vi "setUp.vi"(8 "error in (no error)":errorcluster, 11 "reference in":refnum<class "Telemetry System Tests.lvclass">) -> (0 "error out":errorcluster, 3 "reference out":refnum<class "Telemetry System Tests.lvclass">)   [LabVIEW 2019, in "Telemetry System Tests.lvclass"]
doc: "setUp runs prior to the test method during test execution. Use this method to initialize any object data required by your tests."
uses:
  Telemetry System Tests.lvclass
  C:/Program Files (x86)/National Instruments/LabVIEW 2019/vi.lib/addons/_JKI Toolkits/VI Tester/TestCase.llb/TestCase.lvclass
  Telemetry System Tests.lvclass/Telemetry System Tests.ctl
  <vilib>/addons/_JKI Toolkits/VI Tester/TestCase.llb/TestCase.lvclass
  Telemetry Test Utilities/Telemetry Test Utilities.lvlib
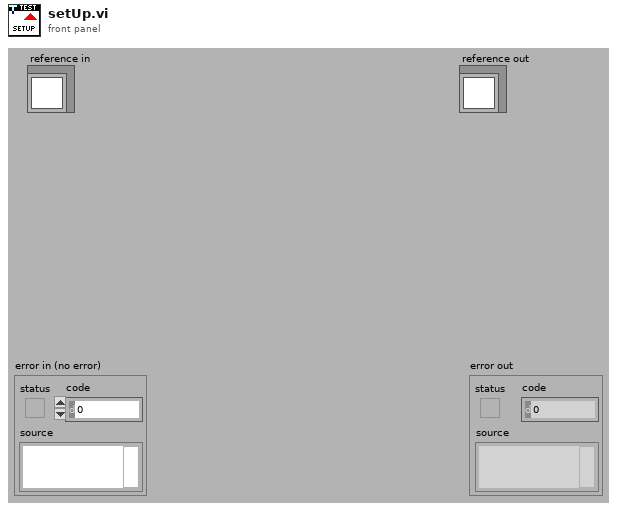
[diagram p1: front panel]
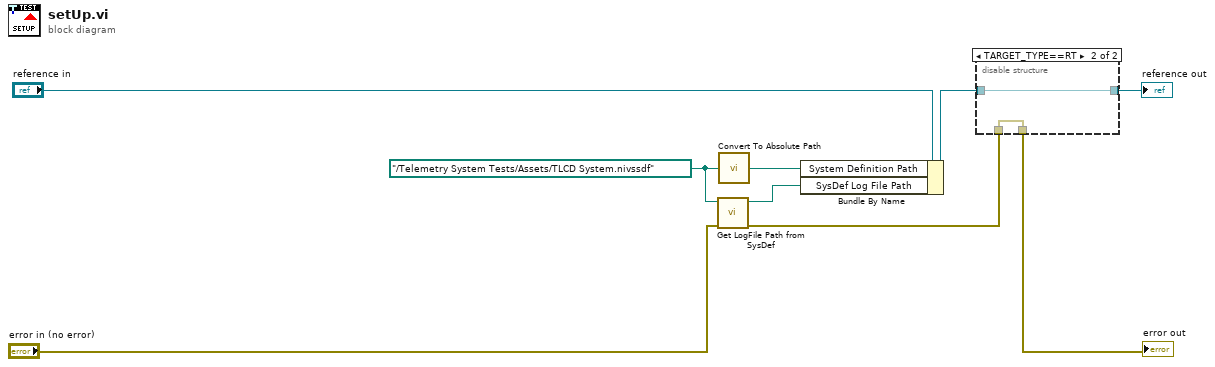
[diagram p0: block diagram]
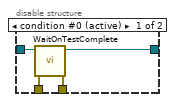
[diagram p2: hidden frame]
diagram:
  w4 = path "../Telemetry System Tests/Assets/TLCD System.nivssdf" ("relative base path")
  n1 = call "Get LogFile Path from SysDef.vi"("error in (no error)"="error in (no error)", "System Definition File"=w4) -> ("error out"=w1:errorcluster, "Log File Path"=w3:path)  [unwired: 8 in]
  n2 = call "Convert To Absolute Path.vi"("System Definition File Path"=w4) -> ("Absolute path"=w5:path)
  n3 = Bundle By Name(cluster="reference in", "System Definition Path"=w5, "SysDef Log File Path"=w3) -> (w6:refnum<class "Telemetry System Tests.lvclass">)
  n4 = disable-structure shown="TARGET_TYPE==RT" {
    disable-tunnel: w1 -> [w13 w14]
    disable-tunnel: [w12 w14] -> w9
    disable-tunnel: [w11 w15] -> w7
    disable-tunnel: w6 -> [w10 w15]
    frame condition #0 (active) {
      n5 = call <vilib>:"WaitOnTestComplete.vi"("error in (no error)"=w13, "TestCase in"=w10) -> ("error out"=w12:errorcluster, "TestCase out"=w11:refnum<class "Telemetry System Tests.lvclass">)  [unwired: 8 in]
    }
    frame condition #1 {
    }
  }
  "error out" <- w9
  "reference out" <- w7
